vi "Second Ex.vi"() -> ()   [LabVIEW 2016]
panel:
  out "Loops":i32
  in  "stop":bool
  out "Meter 2":dbl(knob) scale=0.0..10.0
  out "Meter":dbl(knob) scale=0.0..10.0
  out "Boolean 3":bool
  out "Boolean 2":bool
  in  "Boolean":bool
  in  "Knob":dbl(knob) scale=0.0..10.0
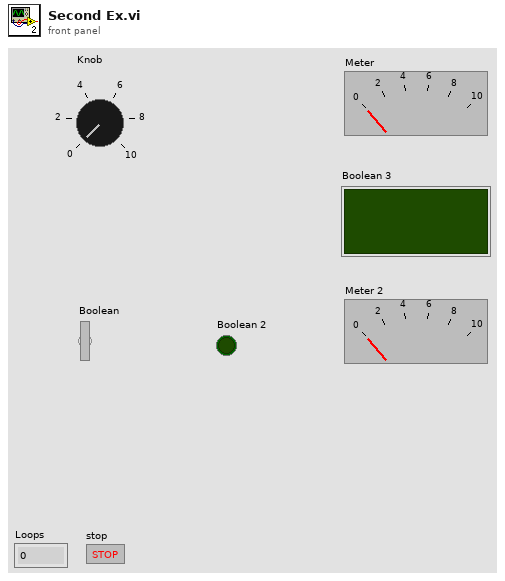
[diagram p1: front panel]
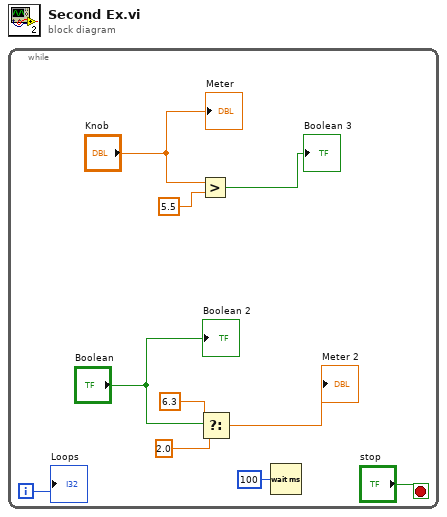
[diagram p0: block diagram]
diagram:
  n1 = while {
    i -> [w2]
    stop <- "stop" stop-if-true
    n2 = Greater?(x="Knob", y=5.5) -> (0:→"Boolean 3":bool)
    n3 = Select(t=6.3, s="Boolean", f=2.0) -> (s? t:f=→"Meter 2":dbl)
    n4 = Wait (ms)(milliseconds to wait=u32 100) -> ()  [unwired: 1 out]
    "Boolean 2" <- "Boolean"
    "Meter" <- "Knob"
    "Loops" <- w2
  }
